vi "LabVIEW_MQTT_Toolkit_V2.vi"() -> ()   [LabVIEW 2021] (continued)
                w5573 = T14 2 items=["User Home"=0, "User Desktop"=1, "User Documents"=2, "User Application Data"=3, "User Preferences"=4, "User Temporary"=5, "Public Documents"=6, "Public Application Data"=7, "Public Preferences"=8, "Public Cache"=13, "System Core Libraries"=9, "System Installed Libraries"=10, "Application Files"=11, "Boot Volume Root"=12] ("system directory type")
                n2249 = Search and Replace String(replace all?=TRUE ("replace all? (F)"), input string=w5568, search string="/") -> (result string=w5589:string)  [unwired: 5 in, 3 out]
                n2250 = Concatenate Strings(w5566, "TimeStamp;Measure Ch_X(g);Ch_Y(g);INC_X(Deg);INC_Y(Deg)", "\n") -> (w5582:string)
                n2251 = Concatenate Strings(w5589, "_" ("string"), "S_E_T.csv") -> (w5590:string)
                n2252 = call <vilib>:"Get System Directory.vi"("system directory type"=w5573) -> ("system directory"=w5583:path)  [unwired: 10 in]
                n2253 = Decimate 1D Array(w5606) -> (w5605:dbl[], w5603:dbl[], w5601:dbl[], w5602:dbl[])
                n2254 = for {
                  tunnel: [w5637] -> w5600 mode=indexing
                  tunnel: w5604 -> [w5631] mode=indexing
                  tunnel: w5605 -> [w5628] mode=indexing
                  tunnel: w5603 -> [w5627] mode=indexing
                  tunnel: w5601 -> [w5626] mode=indexing
                  tunnel: w5602 -> [w5625] mode=indexing
                  tunnel: [w5628] -> w5599 mode=indexing
                  tunnel: [w5627] -> w5598 mode=indexing
                  tunnel: [w5626] -> w5597 mode=indexing
                  tunnel: [w5625] -> w5596 mode=indexing
                  tunnel: w5595 -> [w5620]
                  tunnel: w5594 -> [w5619]
                  tunnel: w5593 -> [w5618] mode=indexing
                  tunnel: w5592 -> [w5617]
                  tunnel: [w5612] -> w5591
                  n2255 = Join Numbers(hi=w5620, lo=w5619) -> ((hi.lo)=w5622:u32)
                  n2256 = To Double Precision Float(number=w5618) -> (double precision float=w5623:dbl)
                  n2257 = Number To Decimal String(number=w5631) -> (decimal integer string=w5636:string)  [unwired: 1 in]
                  n2258 = Number To Fractional String(number=w5628, precision (6)=i16 3 ("width (-)")) -> (F-format string=w5638:string)  [unwired: 2 in]
                  n2259 = Number To Fractional String(number=w5627, precision (6)=i16 3 ("width (-)")) -> (F-format string=w5634:string)  [unwired: 2 in]
                  n2260 = Number To Fractional String(number=w5626, precision (6)=i16 3 ("width (-)")) -> (F-format string=w5632:string)  [unwired: 2 in]
                  n2261 = Number To Fractional String(number=w5625, precision (6)=i16 3 ("width (-)")) -> (F-format string=w5629:string)  [unwired: 2 in]
                  n2262 = Build Array(w5636, w5638, w5634, w5632, w5629) -> (w5637:string[])
                  n2263 = Divide(x=w5623, y=w5617) -> (x/y=w5624:dbl)
                  n2264 = To Unsigned Quad Integer(1:w5622) -> (0:w5621:u64)
                  n2265 = call "Unix Time to Timestamp.vi"("Fractional Second"=w5624, "Unix Time (s)"=w5621) -> ("Timestamp"=w5611:timestamp)  [unwired: 8 in, 1 out]
                  n2266 = Format Date/Time String(seconds (now)=w5611, UTC format=TRUE) -> (date/time string=w5613:string)  [unwired: 1 in]
                  n2267 = Scan From String(format string="%<%x %H:%M:%S%3u>T", input string=w5613) -> (output 1=w5614:timestamp)  [unwired: 3 in, 3 out]
                  n2268 = To Double Precision Float(number=w5614) -> (double precision float=w5612:dbl)
                }
                n2269 = Build Path(base path=w5583, name or relative path="Logfile") -> (appended path=w5584:path)
                n2270 = call <vilib>:"Check if File or Folder Exists.vi"("path"=w5584) -> ("file or folder exists?"=w5585:bool, "dup path"=w5586:path)  [unwired: 8 in, 1 out]
                n2271 = case shown="False" w5585 {
                  tunnel: w5586 -> [w5609 w5610]
                  tunnel: [w5608 w5610] -> w5587
                  frame False {
                    n2272 = Create Folder(path (use dialog)=w5609) -> (created path=w5608:path)  [unwired: 2 in, 2 out]
                  }
                  frame True {
                  }
                }
                n2273 = Build Path(base path=w5587, name or relative path=w5590) -> (appended path=w5588:path)
                n2274 = Open/Create/Replace File(file path (use dialog)=w5588, operation (0:open)=T11."open or create") -> (refnum out=w5581:refnum<file>, error out=w5579:errorcluster)  [unwired: 4 in, 1 out]
                n2275 = Write to Text File(file (use dialog)=w5581, text=w5582, error in=w5579) -> (refnum out=w5580:refnum<file>, error out=w5578:errorcluster)  [unwired: 1 in, 1 out]
                n2276 = Close File(refnum=w5580, error in=w5578) -> (path=w5567:path)  [unwired: 1 out]
              }
              frame 31 {
                w5647 = T14 2 items=["User Home"=0, "User Desktop"=1, "User Documents"=2, "User Application Data"=3, "User Preferences"=4, "User Temporary"=5, "Public Documents"=6, "Public Application Data"=7, "Public Preferences"=8, "Public Cache"=13, "System Core Libraries"=9, "System Installed Libraries"=10, "Application Files"=11, "Boot Volume Root"=12] ("system directory type")
                n2277 = Search and Replace String(replace all?=TRUE ("replace all? (F)"), input string=w5642, search string="/") -> (result string=w5663:string)  [unwired: 5 in, 3 out]
                n2278 = Concatenate Strings(w5640, "TimeStamp;Measure Ch_Z(g);Ch_X(g);Ch_Y(g);INC_X(Deg);INC_Y(Deg)", "\n") -> (w5656:string)
                n2279 = Concatenate Strings(w5663, "_" ("string"), "S_E_T.csv") -> (w5664:string)
                n2280 = call <vilib>:"Get System Directory.vi"("system directory type"=w5647) -> ("system directory"=w5657:path)  [unwired: 10 in]
                n2281 = Decimate 1D Array(w5682) -> (w5681:dbl[], w5680:dbl[], w5679:dbl[], w5678:dbl[], w5676:dbl[])
                n2282 = for {
                  tunnel: [w5716] -> w5675 mode=indexing
                  tunnel: w5677 -> [w5710] mode=indexing
                  tunnel: w5681 -> [w5705] mode=indexing
                  tunnel: w5680 -> [w5704] mode=indexing
                  tunnel: w5679 -> [w5703] mode=indexing
                  tunnel: w5678 -> [w5702] mode=indexing
                  tunnel: w5676 -> [w5701] mode=indexing
                  tunnel: [w5705] -> w5674 mode=indexing
                  tunnel: [w5704] -> w5673 mode=indexing
                  tunnel: [w5703] -> w5672 mode=indexing
                  tunnel: [w5702] -> w5671 mode=indexing
                  tunnel: [w5701] -> w5670 mode=indexing
                  tunnel: w5669 -> [w5696]
                  tunnel: w5668 -> [w5695]
                  tunnel: w5667 -> [w5694] mode=indexing
                  tunnel: w5666 -> [w5693]
                  tunnel: [w5687] -> w5665
                  n2283 = Join Numbers(hi=w5696, lo=w5695) -> ((hi.lo)=w5698:u32)
                  n2284 = To Double Precision Float(number=w5694) -> (double precision float=w5699:dbl)
                  n2285 = Number To Decimal String(number=w5710) -> (decimal integer string=w5715:string)  [unwired: 1 in]
                  n2286 = Number To Fractional String(number=w5705, precision (6)=i16 3 ("width (-)")) -> (F-format string=w5717:string)  [unwired: 2 in]
                  n2287 = Number To Fractional String(number=w5704, precision (6)=i16 3 ("width (-)")) -> (F-format string=w5713:string)  [unwired: 2 in]
                  n2288 = Number To Fractional String(number=w5703, precision (6)=i16 3 ("width (-)")) -> (F-format string=w5711:string)  [unwired: 2 in]
                  n2289 = Number To Fractional String(number=w5702, precision (6)=i16 3 ("width (-)")) -> (F-format string=w5708:string)  [unwired: 2 in]
                  n2290 = Number To Fractional String(number=w5701, precision (6)=i16 3 ("width (-)")) -> (F-format string=w5706:string)  [unwired: 2 in]
                  n2291 = Build Array(w5715, w5717, w5713, w5711, w5708, w5706) -> (w5716:string[])
                  n2292 = Divide(x=w5699, y=w5693) -> (x/y=w5700:dbl)
                  n2293 = To Unsigned Quad Integer(1:w5698) -> (0:w5697:u64)
                  n2294 = call "Unix Time to Timestamp.vi"("Fractional Second"=w5700, "Unix Time (s)"=w5697) -> ("Timestamp"=w5688:timestamp)  [unwired: 8 in, 1 out]
                  n2295 = Format Date/Time String(seconds (now)=w5688, UTC format=TRUE) -> (date/time string=w5689:string)  [unwired: 1 in]
                  n2296 = Scan From String(format string="%<%x %H:%M:%S%3u>T", input string=w5689) -> (output 1=w5690:timestamp)  [unwired: 3 in, 3 out]
                  n2297 = To Double Precision Float(number=w5690) -> (double precision float=w5687:dbl)
                }
                n2298 = Build Path(base path=w5657, name or relative path="Logfile") -> (appended path=w5658:path)
                n2299 = call <vilib>:"Check if File or Folder Exists.vi"("path"=w5658) -> ("file or folder exists?"=w5659:bool, "dup path"=w5660:path)  [unwired: 8 in, 1 out]
                n2300 = case shown="False" w5659 {
                  tunnel: w5660 -> [w5685 w5686]
                  tunnel: [w5684 w5686] -> w5661
                  frame False {
                    n2301 = Create Folder(path (use dialog)=w5685) -> (created path=w5684:path)  [unwired: 2 in, 2 out]
                  }
                  frame True {
                  }
                }
                n2302 = Build Path(base path=w5661, name or relative path=w5664) -> (appended path=w5662:path)
                n2303 = Open/Create/Replace File(file path (use dialog)=w5662, operation (0:open)=T11."open or create") -> (refnum out=w5655:refnum<file>, error out=w5653:errorcluster)  [unwired: 4 in, 1 out]
                n2304 = Write to Text File(file (use dialog)=w5655, text=w5656, error in=w5653) -> (refnum out=w5654:refnum<file>, error out=w5652:errorcluster)  [unwired: 1 in, 1 out]
                n2305 = Close File(refnum=w5654, error in=w5652) -> (path=w5641:path)  [unwired: 1 out]
              }
            }
            "Enabled channels" <- w3579
            "CH_Z Graph" <- w3501
            "CH_X Graph" <- w3499
            "CH_Y Graph" <- w3498
            "INC_X Graph" <- w3497
            "INC_Y Graph" <- w3496
            "File path" <- w3488
            n2306 = property on="CH_Z Graph" class="WFChart (strict)"("XScale.Offset"=w3491) -> ()  [unwired: 2 in, 2 out]
            n2307 = property on="INC_Y Graph" class="WFChart (strict)"("XScale.Offset"=w3487) -> ()  [unwired: 2 in, 2 out]
            n2308 = property on="CH_Y Graph" class="WFChart (strict)"("XScale.Offset"=w3490) -> ()  [unwired: 2 in, 2 out]
            n2309 = property on="CH_X Graph" class="WFChart (strict)"("XScale.Offset"=w3441) -> ()  [unwired: 2 in, 2 out]
            n2310 = property on="INC_X Graph" class="WFChart (strict)"("XScale.Offset"=w3489) -> ()  [unwired: 2 in, 2 out]
            n2311 = call-poly <vilib>:"Write Delimited Spreadsheet.vi"("file path (dialog if empty)"=w3488, "format (%s)"="%s", "2D data"=w3503, "append to file? (new file:F)"=TRUE, "transpose? (no:F)"=FALSE, "delimiter (\\t)"=";" ("delimiter (\\t)")) -> ()  [unwired: 8 in, 2 out]
          }
          frame 7 {
            w5764 = "NA"
            w5800 = T14 2 items=["User Home"=0, "User Desktop"=1, "User Documents"=2, "User Application Data"=3, "User Preferences"=4, "User Temporary"=5, "Public Documents"=6, "Public Application Data"=7, "Public Preferences"=8, "Public Cache"=13, "System Core Libraries"=9, "System Installed Libraries"=10, "Application Files"=11, "Boot Volume Root"=12] ("system directory type")
            # "function to write data in log file"
            # "this block conttain measures + dates of different  sensor channels"
            # "logfile path"
            # "logfile headers"
            # "this block contain Channels bitmap"
            n2312 = String To Byte Array(string=w5907) -> (unsigned byte array=w5841:u8[])
            n2313 = property on="Measure mode" class="Str"() -> ("Value"=w5730:string)  [unwired: 2 in, 2 out]
            n2314 = Array Size(array=w5841) -> (size(s)=w5843:i32)
            n2315 = Array To Cluster(array=w5841) -> (cluster=w5906:T18)
            n2316 = Subtract(x=w5843, y=35) -> (x-y=w5842:i32)
            n2317 = call <vilib>:"Get System Directory.vi"("system directory type"=w5800) -> ("system directory"=w5807:path)  [unwired: 10 in]
            n2318 = String Subset(string=w5755, offset (0)=0, length (rest)=16 ("length (rest)")) -> (substring=w5754:string)
            n2319 = Equal?(x=w5730, y="S_E_T") -> (x = y?=w5732:bool)
            n2320 = Array Subset(array=w5841, index=36, length=w5842) -> (w5743:u8[])
            n2321 = property on="concatenated string" class="Str"() -> ("Value"=w5729:string)  [unwired: 2 in, 2 out]
            n2322 = property on="Measure mode" class="Str"() -> ("Value"=w5726:string)  [unwired: 2 in, 2 out]
            n2323 = Unbundle(w5906) -> ("unsigned byte array[2]"=w5749:u8, "unsigned byte array[3]"=w5905:u8, "unsigned byte array[4]"=w5904:u8, "unsigned byte array[5]"=w5898:u8, "unsigned byte array[6]"=w5897:u8, "unsigned byte array[7]"=w5896:u8, "unsigned byte array[8]"=w5895:u8, "unsigned byte array[9]"=w5894:u8, "unsigned byte array[10]"=w5893:u8, "unsigned byte array[12]"=w5892:u8, "unsigned byte array[16]"=w5889:u8, "unsigned byte array[17]"=w5886:u8, "unsigned byte array[18]"=w5885:u8, "unsigned byte array[19]"=w5873:u8, "unsigned byte array[20]"=w5884:u8, "unsigned byte array[21]"=w5883:u8, "unsigned byte array[22]"=w5882:u8, "unsigned byte array[23]"=w5881:u8, "unsigned byte array[24]"=w5880:u8, "unsigned byte array[25]"=w5890:u8, "unsigned byte array[26]"=w5879:u8, "unsigned byte array[27]"=w5878:u8, "unsigned byte array[28]"=w5871:u8, "unsigned byte array[29]"=w5877:u8, "unsigned byte array[30]"=w5876:u8, "unsigned byte array[31]"=w5875:u8, "unsigned byte array[32]"=w5891:u8, "unsigned byte array[33]"=w5874:u8, "unsigned byte array[34]"=w5887:u8, "unsigned byte array[35]"=w5888:u8)  [unwired: 6 out]
            n2324 = Join Numbers(hi=w5904, lo=w5905) -> ((hi.lo)=w5903:u16)
            n2325 = Join Numbers(hi=w5897, lo=w5898) -> ((hi.lo)=w5902:u16)
            n2326 = Join Numbers(hi=w5894, lo=w5895) -> ((hi.lo)=w5900:u16)
            n2327 = Join Numbers(hi=w5886, lo=w5889) -> ((hi.lo)=w5872:u16)
            n2328 = Join Numbers(hi=w5880, lo=w5881) -> ((hi.lo)=w5866:u16)
            n2329 = Join Numbers(hi=w5879, lo=w5890) -> ((hi.lo)=w5870:u16)
            n2330 = Join Numbers(hi=w5874, lo=w5891) -> ((hi.lo)=w5867:u16)
            n2331 = Join Numbers(hi=w5888, lo=w5887) -> ((hi.lo)=w5741:u16)
            "Number of data per channel" <- w5741
            n2332 = To Unsigned Byte Integer(number=w5892) -> (unsigned 8bit integer=w5753:u8)
            n2333 = case shown="1001" w5753 {
              tunnel: ["" "no active channel" "chZ " "chX " "chZ & chX " "chY " "chZ & chY  " "chX & chY " "chZ& chX& chY " "INC_X " "chZ & INC_X " "chX & INC_X " "chZ& chX & INC_X " "chY & INC_X " "chZ  & chY & INC_X " "chX  & chY & INC_X " "chZ& chX  & chY & INC_X " "INC_Y  " " chZ & INC_Y " " chX & INC_Y  " "chZ & chX & INC_Y " " chY & INC_Y " "chZ & chY & INC_Y" "chX & chY & INC_Y" " chZ &chX & chY & INC_Y  " " INC_X & INC_Y " "chZ &   INC_X & INC_Y" "chX & INC_X & INC_Y" " chZ & chX &  INC_X & INC_Y  " " chY &  INC_X & INC_Y  " "chZ & chY &  INC_X & INC_Y " "chX & chY &  INC_X & INC_Y" "chZ & chX & chY &  INC_X & INC_Y"] -> w5752
              frame Default {
              }
              frame 0 {
              }
              frame 1 {
              }
              frame 2 {
              }
              frame 3 {
              }
              frame 4 {
              }
              frame 5 {
              }
              frame 6 {
              }
              frame 7 {
              }
              frame 8 {
              }
              frame 9 {
              }
              frame 10 {
              }
              frame 11 {
              }
              frame 12 {
              }
              frame 13 {
              }
              frame 14 {
              }
              frame 15 {
              }
              frame 16 {
              }
              frame 17 {
              }
              frame 18 {
              }
              frame 19 {
              }
              frame 20 {
              }
              frame 21 {
              }
              frame 22 {
              }
              frame 23 {
              }
              frame 24 {
              }
              frame 25 {
              }
              frame 26 {
              }
              frame 27 {
              }
              frame 28 {
              }
              frame 29 {
              }
              frame 30 {
              }
              frame 31 {
              }
            }
            "Enabled channels" <- w5752
            n2334 = Join Numbers(hi=w5893, lo=w5900) -> ((hi.lo)=w5899:u32)
            n2335 = Join Numbers(hi=w5896, lo=w5902) -> ((hi.lo)=w5901:u32)
            n2336 = To Word Integer(number=w5903) -> (16bit integer=w5742:i16)
            "Acquisition frequency" <- w5742
            n2337 = To Long Integer(number=w5901) -> (32bit integer=→"Acquisition cycle":i32)
            n2338 = Format Into String(format string="%02d/%02d/%d %02d:%02d:%02d,%d", w5873, w5885, w5872, w5884, w5883, w5882, w5866) -> (resulting string=w5722:string)  [unwired: 2 in, 1 out]
            "Start date" <- w5722
            n2339 = Format Into String(format string="%02d/%02d/%d %02d:%02d:%02d,%d", w5871, w5878, w5870, w5877, w5876, w5875, w5867) -> (resulting string=w5719:string)  [unwired: 2 in, 1 out]
            "End date" <- w5719
            n2340 = Equal?(x=w5726, y="Shock Detection ") -> (x = y?=w5727:bool)
            n2341 = Select(t=w5730, s=w5732, f=w5729) -> (s? t:f=w5725:string)
            n2342 = To Long Integer(number=w5899) -> (32bit integer=→"Acquisition duration":i32)
            n2343 = Build Path(base path=w5807, name or relative path="Logfile") -> (appended path=w5808:path)
            n2344 = call <vilib>:"Check if File or Folder Exists.vi"("path"=w5808) -> ("file or folder exists?"=w5809:bool, "dup path"=w5810:path)  [unwired: 8 in, 1 out]
            n2345 = case shown="False" w5809 {
              tunnel: w5810 -> [w5952 w5953]
              tunnel: [w5951 w5953] -> w5811
              frame False {
                n2346 = Create Folder(path (use dialog)=w5952) -> (created path=w5951:path)  [unwired: 2 in, 2 out]
              }
              frame True {
              }
            }
            n2347 = case shown="7" w5749 {
              tunnel: ["" "LDCDA mode" "Alarm mode" "Streaming mode" "S.E.T mode " "Dynamic mode"] -> w5748
              frame Default {
              }
              frame 1 {
              }
              frame 2 {
              }
              frame 3 {
              }
              frame 6 {
              }
              frame 7 {
              }
            }
            "Acquisition Mode" <- w5748
            n2348 = Select(t=w5726, s=w5727, f=w5725) -> (s? t:f=w5724:string)
            n2349 = Concatenate Strings("Start Date;End Date;Ch_Z_Min value date;Ch_Z_Min value;Ch_Z_Max value date;Ch_Z_Max value;Ch_Z_Average value;Ch_X_Min value date;Ch_X_Min value;Ch_X_Max value date;Ch_X_Max value;Ch_X_Average value;Ch_Y_Min value date;Ch_Y_Min value;Ch_Y_Max value date;Ch_Y_Max value;Ch_Y_Average value;INC_X_Min value date;INC_X_Min value_Deg;INC_X_Max value date;INC_X_Max value_Deg;INC_X_Average value_Deg;INC_Y_Min value date\t;INC_Y_Min value_Deg;INC_Y_Max value date;INC_Y_Max value_Deg;INC_Y_Average value\t", "\n") -> (w5806:string)
            n2350 = Concatenate Strings(w5754, "_" ("string"), w5724, "_" ("string"), "Transmit_Math_Mode.txt") -> (w5813:string)
            n2351 = Build Path(base path=w5811, name or relative path=w5813) -> (appended path=w5812:path)
            n2352 = Open/Create/Replace File(file path (use dialog)=w5812, operation (0:open)=T11."open or create") -> (refnum out=w5805:refnum<file>, error out=w5803:errorcluster)  [unwired: 4 in, 1 out]
            n2353 = Write to Text File(file (use dialog)=w5805, text=w5806, error in=w5803) -> (refnum out=w5804:refnum<file>, error out=w5802:errorcluster)  [unwired: 1 in, 1 out]
            n2354 = Close File(refnum=w5804, error in=w5802) -> (path=w5796:path)  [unwired: 1 out]
            "File path" <- w5796
            n2355 = Decimate 1D Array(w5743) -> (w5865:u8[], w5864:u8[], w5863:u8[], w5862:u8[], w5861:u8[], w5860:u8[], w5859:u8[], w5858:u8[], w5857:u8[], w5856:u8[], w5855:u8[], w5854:u8[], w5853:u8[], w5852:u8[], w5851:u8[], w5850:u8[], w5849:u8[], w5848:u8[], w5847:u8[], w5846:u8[], w5845:u8[])
            n2356 = for {
              tunnel: w5741 -> [w5988]
              tunnel: w5865 -> [w6021] mode=indexing
              tunnel: w5864 -> [w6020] mode=indexing
              tunnel: w5863 -> [w6019] mode=indexing
              tunnel: w5862 -> [w6018] mode=indexing
              tunnel: w5861 -> [w6017] mode=indexing
              tunnel: w5860 -> [w6016] mode=indexing
              tunnel: w5859 -> [w6015] mode=indexing
              tunnel: w5858 -> [w6014] mode=indexing
              tunnel: w5857 -> [w5978] mode=indexing
              tunnel: w5856 -> [w6013] mode=indexing
              tunnel: w5855 -> [w6012] mode=indexing
              tunnel: w5854 -> [w6011] mode=indexing
              tunnel: w5853 -> [w6010] mode=indexing
              tunnel: w5852 -> [w6009] mode=indexing
              tunnel: w5851 -> [w6008] mode=indexing
              tunnel: w5850 -> [w6007] mode=indexing
              tunnel: w5849 -> [w6006] mode=indexing
              tunnel: w5848 -> [w5976] mode=indexing
              tunnel: w5847 -> [w6005] mode=indexing
              tunnel: w5846 -> [w6004] mode=indexing
              tunnel: w5845 -> [w5977] mode=indexing
              tunnel: [w5964] -> w5829 mode=indexing
              tunnel: [w6003] -> w5830 mode=indexing
              tunnel: [w5965] -> w5838 mode=indexing
              tunnel: w5722 -> [w5960]
              tunnel: w5742 -> [w5990]
              tunnel: [w5966] -> w5836 mode=indexing
              tunnel: [w5970] -> w5833 mode=indexing
              tunnel: w5722 -> [w5957]
              tunnel: w5719 -> [w5956]
              tunnel: [w5955] -> w5721
              n2357 = Join Numbers(hi=w6018, lo=w6019) -> ((hi.lo)=w6033:u16)
              n2358 = Join Numbers(hi=w6020, lo=w6021) -> ((hi.lo)=w6034:u16)
              n2359 = Join Numbers(hi=w6010, lo=w6011) -> ((hi.lo)=w6030:u16)
              n2360 = Join Numbers(hi=w6012, lo=w6013) -> ((hi.lo)=w6031:u16)
              n2361 = Join Numbers(hi=w6006, lo=w6007) -> ((hi.lo)=w5982:u16)
              n2362 = Join Numbers(hi=w6004, lo=w6005) -> ((hi.lo)=w6029:u16)
              n2363 = Sign(1:w5978) -> (0:w6032:u8)
              n2364 = To Byte Integer(number=w6014) -> (8bit integer=w5974:i8)
              n2365 = To Byte Integer(number=w6015) -> (8bit integer=w5975:i8)
              n2366 = Sign(1:w5976) -> (0:w5981:u8)
              n2367 = Sign(1:w5977) -> (0:w6028:u8)
              n2368 = Join Numbers(hi=w6016, lo=w6017) -> ((hi.lo)=w6026:u16)
              "index minval" <- w6026
              n2369 = Join Numbers(hi=w6008, lo=w6009) -> ((hi.lo)=w6022:u16)
              "index maxval" <- w6022
              n2370 = Concatenate Strings(w5957, ";", w5956) -> (w5955:string)
              n2371 = Join Numbers(hi=w5974, lo=w5975) -> ((hi.lo)=w5987:u16)
              n2372 = Join Numbers(hi=w6033, lo=w6034) -> ((hi.lo)=w6027:u32)
              "fid min ch1" <- w6027
              n2373 = Join Numbers(hi=w6030, lo=w6031) -> ((hi.lo)=w6023:u32)
              "fid max ch1" <- w6023
              n2374 = To Byte Integer(number=w5981) -> (8bit integer=w5979:i8)
              n2375 = To Word Integer(number=w5982) -> (16bit integer=w5983:i16)
              n2376 = To Byte Integer(number=w6028) -> (8bit integer=w5985:i8)
              n2377 = To Word Integer(number=w6029) -> (16bit integer=w5984:i16)
              n2378 = Scan From String(format string="%<%x %H:%M:%S%3u>T", input string=w5960) -> (output 1=w5995:timestamp)  [unwired: 3 in, 3 out]
              n2379 = Multiply(x=w5988, y=w6027) -> (x*y=w6025:u32)
              n2380 = Multiply(x=w5988, y=w6023) -> (x*y=w6024:u32)
              n2381 = case shown="1" w5979 {
                tunnel: w5983 -> [_ w6043 w6049]
                tunnel: [_ w6041 w6048] -> w5964
                frame Default {
                }
                frame 1 {
                  n2382 = Equal?(x=w6043, y=i16 0) -> (x = y?=w6045:bool)
                  n2383 = Divide(x=w6043, y=-1000.0) -> (x/y=w6042:dbl)
                  n2384 = Select(t=0.0 ("f"), s=w6045, f=w6042) -> (s? t:f=w6041:dbl)
                }
                frame 0 {
                  n2385 = Equal?(x=w6049, y=i16 -1) -> (x = y?=w6052:bool)
                  n2386 = Divide(x=w6049, y=1000.0) -> (x/y=w6050:dbl)
                  n2387 = Select(t=0.0 ("f"), s=w6052, f=w6050) -> (s? t:f=w6048:dbl)
                }
              }
              n2388 = case shown="0" w5985 {
                tunnel: [_ w6036 w6039] -> w6003
                tunnel: w5984 -> [_ w6035 w6038]
                frame Default {
                }
                frame 1 {
                  n2389 = Divide(x=w6035, y=-1000.0) -> (x/y=w6036:dbl)
                }
                frame 0 {
                  n2390 = Divide(x=w6038, y=1000.0) -> (x/y=w6039:dbl)
                }
              }
              n2391 = To Byte Integer(number=w6032) -> (8bit integer=w5980:i8)
              n2392 = To Word Integer(number=w5987) -> (16bit integer=w5986:i16)
              n2393 = case shown="0" w5980 {
                tunnel: w5986 -> [_ w6060 w6065]
                tunnel: [_ w6057 w6064] -> w5965
                frame Default {
                }
                frame 1 {
                  n2394 = Equal?(x=w6060, y=i16 -1) -> (x = y?=w6058:bool)
                  n2395 = Divide(x=w6060, y=-1000.0) -> (x/y=w6055:dbl)
                  n2396 = Select(t=0.0 ("f"), s=w6058, f=w6055) -> (s? t:f=w6057:dbl)
                }
                frame 0 {
                  n2397 = Equal?(x=w6065, y=i16 -1) -> (x = y?=w6066:bool)
                  n2398 = Divide(x=w6065, y=1000.0) -> (x/y=w6062:dbl)
                  n2399 = Select(t=0.0 ("f"), s=w6066, f=w6062) -> (s? t:f=w6064:dbl)
                }
              }
              n2400 = Add(x=w6026, y=w6025) -> (x+y=w5992:u32)
              n2401 = Add(x=w6022, y=w6024) -> (x+y=w5994:u32)
              n2402 = Divide(x=1, y=w5990) -> (x/y=w5997:dbl)
              n2403 = Divide(x=1, y=w5990) -> (x/y=w6000:dbl)
              n2404 = Multiply(x=w5997, y=w5992) -> (x*y=w5998:dbl)
              n2405 = Multiply(x=w6000, y=w5994) -> (x*y=w6001:dbl)
              n2406 = call "Timestamp to Unix Time.vi"("Timestamp (now)"=w5995) -> ("Unix Time (s)"=w6002:i64)  [unwired: 9 in, 1 out]
              n2407 = Add(x=w6002, y=w5998) -> (x+y=w5996:dbl)
              n2408 = Add(x=w6002, y=w6001) -> (x+y=w5999:dbl)
              n2409 = call "Unix Time to Timestamp.vi"("Unix Time (s)"=w5996) -> ("Timestamp"=w5973:timestamp)  [unwired: 9 in, 1 out]
              n2410 = call "Unix Time to Timestamp.vi"("Unix Time (s)"=w5999) -> ("Timestamp"=w5967:timestamp)  [unwired: 9 in, 1 out]
              n2411 = Format Date/Time String(seconds (now)=w5973, UTC format=TRUE) -> (date/time string=w5971:string)  [unwired: 1 in]
              n2412 = Format Date/Time String(seconds (now)=w5967, UTC format=TRUE) -> (date/time string=w5968:string)  [unwired: 1 in]
              n2413 = Equal To 0?(x=w5964) -> (x = 0?=w5962:bool)
              n2414 = Equal To 0?(x=w5965) -> (x = 0?=w5963:bool)
              n2415 = And(x=w5963, y=w5962) -> (x .and. y?=w5961:bool)
              n2416 = Select(t="NA", s=w5961, f=w5971) -> (s? t:f=w5970:string)
              n2417 = Select(t="NA", s=w5961, f=w5968) -> (s? t:f=w5966:string)
            }
            "Max value" <- w5829
            "Average value" <- w5830
            "Min value" <- w5838
            "Min date" <- w5833
            "Max date" <- w5836
            n2418 = Equal?(x=w5793, y=u8 1) -> (x = y?=w5744:bool)
            n2419 = Array To Cluster(array=w5833) -> (cluster=w5834:T19)
            n2420 = Array To Cluster(array=w5838) -> (cluster=w5837:T20)
            n2421 = Array To Cluster(array=w5836) -> (cluster=w5835:T19)
            n2422 = Array To Cluster(array=w5829) -> (cluster=w5832:T20)
            n2423 = Array To Cluster(array=w5830) -> (cluster=w5831:T20)
            n2424 = Equal?(x=w5793, y=u8 6) -> (x = y?=w5720:bool)
            n2425 = Unbundle(w5834) -> ("[0]"=w5740:string, "[1]"=w5825:string, "[2]"=w5822:string, "[3]"=w5738:string, "[4]"=w5737:string)
            n2426 = Unbundle(w5837) -> ("[0]"=w5739:dbl, "[1]"=w5747:dbl, "[2]"=w5821:dbl, "[3]"=w5783:dbl, "[4]"=w5782:dbl)
            n2427 = Unbundle(w5835) -> ("[0]"=w5828:string, "[1]"=w5824:string, "[2]"=w5787:string, "[3]"=w5736:string, "[4]"=w5735:string)
            n2428 = Unbundle(w5832) -> ("[0]"=w5827:dbl, "[1]"=w5820:dbl, "[2]"=w5819:dbl, "[3]"=w5781:dbl, "[4]"=w5780:dbl)
            n2429 = Unbundle(w5831) -> ("[0]"=w5826:dbl, "[1]"=w5823:dbl, "[2]"=w5818:dbl, "[3]"=w5779:dbl, "[4]"=w5778:dbl)
            n2430 = Not Or(1:w5720, 2:w5744) -> (0:w5777:bool)
            n2431 = Number To Fractional String(number=w5783, precision (6)=i16 3 ("width (-)")) -> (F-format string=w5776:string)  [unwired: 2 in]
            n2432 = Number To Fractional String(number=w5781, precision (6)=i16 3 ("width (-)")) -> (F-format string=w5774:string)  [unwired: 2 in]
            n2433 = Number To Fractional String(number=w5779, precision (6)=i16 3 ("width (-)")) -> (F-format string=w5772:string)  [unwired: 2 in]
            n2434 = Number To Fractional String(number=w5782, precision (6)=i16 3 ("width (-)")) -> (F-format string=w5775:string)  [unwired: 2 in]
            n2435 = Number To Fractional String(number=w5780, precision (6)=i16 3 ("width (-)")) -> (F-format string=w5773:string)  [unwired: 2 in]
            n2436 = Number To Fractional String(number=w5778, precision (6)=i16 3 ("width (-)")) -> (F-format string=w5771:string)  [unwired: 2 in]
            n2437 = Select(t=w5737, s=w5777, f="") -> (s? t:f=w5786:string)
            n2438 = Select(t=w5735, s=w5777, f="") -> (s? t:f=w5790:string)
            n2439 = Select(t=w5738, s=w5777, f="NA") -> (s? t:f=w5789:string)
            n2440 = Select(t=w5736, s=w5777, f="NA") -> (s? t:f=w5788:string)
            n2441 = Select(t=w5776, s=w5777, f=w5764) -> (s? t:f=w5770:string)
            n2442 = Select(t=w5774, s=w5777, f=w5764) -> (s? t:f=w5768:string)
            n2443 = Select(t=w5772, s=w5777, f=w5764) -> (s? t:f=w5765:string)
            n2444 = Select(t=w5775, s=w5777, f=w5764) -> (s? t:f=w5769:string)
            n2445 = Select(t=w5773, s=w5777, f=w5764) -> (s? t:f=w5767:string)
            n2446 = Select(t=w5771, s=w5777, f=w5764) -> (s? t:f=w5766:string)
            n2447 = Format Into String(format string=";%S ;%.3f;%s;%.3f;%.3f;%S;%.3f;%s;%.3f;%.3f;%S ;%.3f ;%s;%.3f; %.3f ;%s ;%s; %s ;%s ;%s; %s ;%s ;%s ;%s ;%s\\n", initial string=w5721, w5740, w5739, w5828, w5827, w5826, w5825, w5747, w5824, w5820, w5823, w5822, w5821, w5787, w5819, w5818, w5789, w5770, w5788, w5768, w5765, w5786, w5769, w5790, w5767, w5766) -> (resulting string=w5816:string)  [unwired: 1 in, 1 out]
            n2448 = Build Array(w5816) -> (w5815:string[])
            n2449 = call-poly <vilib>:"Write Delimited Spreadsheet.vi"("file path (dialog if empty)"=w5796, "1D data"=w5815, "append to file? (new file:F)"=TRUE, "transpose? (no:F)"=TRUE, "delimiter (\\t)"=";" ("delimiter (\\t)")) -> ()  [unwired: 9 in, 2 out]
            "Device type" <- w5908
            "String" <- "Ch_Z                    Ch_X                     Ch_Y                     INC_X                     INC_Y" ("String")
          }
        }
        "Measure mode" <- w195
        "Date & time" <- w190
        "Sensor Label" <- w193
        "Device type" <- w194
        "Date & time" <- w190
        "Sensor label" <- w193
        "Measure mode" <- w195
        "Measure" <- w180
        "Measure" <- w180
        "Numeric" <- w175
      }
      event "Data acq .mode": Value Change {
        # "this block is used to disable and enable sampling rate according to the mode of acquisition"
        n2450 = event-data() -> ()  [unwired: 1 in, 1 out]
        n2451 = property on="Data acq .mode" class="Ring (strict)"() -> ("Value"=w6077:u8)  [unwired: 2 in, 2 out]
        n2452 = case shown="3" w6077 {
          tunnel: "Device type" -> [_ w6084 _ w6095 _ _ _]
          frame 2 {
            (unwired) i32[] [1, 2, 3, 4, 5, 6, 7, 8, 9, 10, 11, 12, 13, 14, 15, 16, 17, 18, 19, 20, 21] ("Disabled Items []")
            w6080 = T10."Enabled" ("Disabled")
            w6079 = T10."Disabled and Grayed Out" ("Disabled")
            n2453 = property on="Streaming options" class="RadioBtnsControl (strict)"("DisabledEnum"=w6079) -> ()  [unwired: 2 in, 2 out]
            n2454 = property on="Data Acq duration" class="Clust (strict)"("DisabledEnum"=w6079) -> ()  [unwired: 2 in, 2 out]
            n2455 = property on="Math notif ratio" class="DigNum (strict)"("DisabledEnum"=w6080) -> ()  [unwired: 2 in, 2 out]
            n2456 = property on="Tx ratio" class="DigNum (strict)"("DisabledEnum"=w6080) -> ()  [unwired: 2 in, 2 out]
            n2457 = property on="Data acq cycle/Notif cycle" class="Clust (strict)"("DisabledEnum"=w6080) -> ()  [unwired: 2 in, 2 out]
            n2458 = property on="Sampling rate" class="Ring (strict)"("DisabledEnum"=w6079) -> ()  [unwired: 2 in, 2 out]
          }
          frame 3 {
            w6082 = T10."Enabled" ("Disabled")
            w6083 = T10."Disabled and Grayed Out" ("Disabled")
            n2459 = property on="Tx ratio" class="DigNum (strict)"("DisabledEnum"=w6083) -> ()  [unwired: 2 in, 2 out]
            n2460 = property on="Data Acq duration" class="Clust (strict)"("DisabledEnum"=w6083) -> ()  [unwired: 2 in, 2 out]
            n2461 = property on="Math notif ratio" class="DigNum (strict)"("DisabledEnum"=w6083) -> ()  [unwired: 2 in, 2 out]
            n2462 = property on="Data acq cycle/Notif cycle" class="Clust (strict)"("DisabledEnum"=w6083) -> ()  [unwired: 2 in, 2 out]
            n2463 = case shown="1" w6084 {
              frame Default {
              }
              frame 1 {
                n2464 = property on="Sampling rate" class="Ring (strict)"("Disabled Items []"=i32[] [1, 2, 3, 5, 6, 8, 9, 11, 12, 13, 14, 15, 17, 19, 21]) -> ()  [unwired: 2 in, 2 out]
              }
              frame 2 {
                n2465 = property on="Sampling rate" class="Ring (strict)"("Disabled Items []"=i32[] []) -> ()  [unwired: 2 in, 2 out]
              }
              frame 3 {
                n2466 = property on="Sampling rate" class="Ring (strict)"("Disabled Items []"=i32[] []) -> ()  [unwired: 2 in, 2 out]
              }
              frame 4 {
                n2467 = property on="Sampling rate" class="Ring (strict)"("Disabled Items []"=i32[] []) -> ()  [unwired: 2 in, 2 out]
              }
              frame 5 {
                n2468 = property on="Sampling rate" class="Ring (strict)"("Disabled Items []"=i32[] []) -> ()  [unwired: 2 in, 2 out]
              }
              frame 0 {
                n2469 = property on="Sampling rate" class="Ring (strict)"("Disabled Items []"=i32[] []) -> ()  [unwired: 2 in, 2 out]
              }
            }
            n2470 = property on="Sampling rate" class="Ring (strict)"("DisabledEnum"=w6082) -> ()  [unwired: 2 in, 2 out]
            n2471 = property on="Streaming options" class="RadioBtnsControl (strict)"("DisabledEnum"=w6082) -> ()  [unwired: 2 in, 2 out]
            n2472 = property on="Sampling rate" class="Ring (strict)"("Disabled Items []"=i32[] []) -> ()  [unwired: 2 in, 2 out]
          }
          frame 4 {
            w6092 = T10."Enabled" ("Disabled")
            w6091 = T10."Disabled and Grayed Out" ("Disabled")
            n2473 = property on="Data Acq duration" class="Clust (strict)"("DisabledEnum"=w6091) -> ()  [unwired: 2 in, 2 out]
            n2474 = property on="Streaming options" class="RadioBtnsControl (strict)"("DisabledEnum"=w6091) -> ()  [unwired: 2 in, 2 out]
            n2475 = property on="Sampling rate" class="Ring (strict)"("DisabledEnum"=w6091) -> ()  [unwired: 2 in, 2 out]
            n2476 = property on="Math notif ratio" class="DigNum (strict)"("DisabledEnum"=w6091) -> ()  [unwired: 2 in, 2 out]
            n2477 = property on="Tx ratio" class="DigNum (strict)"("DisabledEnum"=w6092) -> ()  [unwired: 2 in, 2 out]
            n2478 = property on="Data acq cycle/Notif cycle" class="Clust (strict)"("DisabledEnum"=w6092) -> ()  [unwired: 2 in, 2 out]
            n2479 = property on="Sampling rate" class="Ring (strict)"("DisabledEnum"=w6091) -> ()  [unwired: 2 in, 2 out]
          }
          frame 5 {
            w6093 = T10."Enabled" ("Disabled")
            w6094 = T10."Disabled and Grayed Out" ("Disabled")
            n2480 = property on="Tx ratio" class="DigNum (strict)"("DisabledEnum"=w6094) -> ()  [unwired: 2 in, 2 out]
            n2481 = property on="Streaming options" class="RadioBtnsControl (strict)"("DisabledEnum"=w6094) -> ()  [unwired: 2 in, 2 out]
            n2482 = property on="Data acq cycle/Notif cycle" class="Clust (strict)"("DisabledEnum"=w6093) -> ()  [unwired: 2 in, 2 out]
            n2483 = property on="Math notif ratio" class="DigNum (strict)"("DisabledEnum"=w6094) -> ()  [unwired: 2 in, 2 out]
            n2484 = property on="Sampling rate" class="Ring (strict)"("Disabled Items []"=i32[] [14, 15, 16, 17, 18, 19, 20, 21]) -> ()  [unwired: 2 in, 2 out]
            n2485 = property on="Sampling rate" class="Ring (strict)"("DisabledEnum"=w6093) -> ()  [unwired: 2 in, 2 out]
            n2486 = property on="Data Acq duration" class="Clust (strict)"("DisabledEnum"=w6093) -> ()  [unwired: 2 in, 2 out]
            n2487 = case shown="Default" w6095 {
              frame Default {
              }
              frame 1 {
                n2488 = property on="Sampling rate" class="Ring (strict)"("Disabled Items []"=i32[] [1, 2, 3, 5, 6, 8, 9, 11, 12, 13, 14, 15, 16, 17, 18, 19, 20, 21]) -> ()  [unwired: 2 in, 2 out]
              }
              frame 2 {
                n2489 = property on="Sampling rate" class="Ring (strict)"("Disabled Items []"=i32[] [14, 15, 16, 17, 18, 19, 20, 21]) -> ()  [unwired: 2 in, 2 out]
              }
              frame 3 {
                n2490 = property on="Sampling rate" class="Ring (strict)"("Disabled Items []"=i32[] [14, 15, 16, 17, 18, 19, 20, 21]) -> ()  [unwired: 2 in, 2 out]
              }
              frame 4 {
                n2491 = property on="Sampling rate" class="Ring (strict)"("Disabled Items []"=i32[] [14, 15, 16, 17, 18, 19, 20, 21]) -> ()  [unwired: 2 in, 2 out]
              }
              frame 5 {
                n2492 = property on="Sampling rate" class="Ring (strict)"("Disabled Items []"=i32[] [14, 15, 16, 17, 18, 19, 20, 21]) -> ()  [unwired: 2 in, 2 out]
              }
              frame 0 {
                n2493 = property on="Sampling rate" class="Ring (strict)"("Disabled Items []"=i32[] [14, 15, 16, 17, 18, 19, 20, 21]) -> ()  [unwired: 2 in, 2 out]
              }
            }
          }
          frame 6 {
            w6104 = T10."Enabled" ("Disabled")
            w6105 = T10."Disabled and Grayed Out" ("Disabled")
            n2494 = property on="Sampling rate" class="Ring (strict)"("DisabledEnum"=w6104) -> ()  [unwired: 2 in, 2 out]
            n2495 = property on="Math notif ratio" class="DigNum (strict)"("DisabledEnum"=w6105) -> ()  [unwired: 2 in, 2 out]
            n2496 = property on="Data Acq duration" class="Clust (strict)"("DisabledEnum"=w6104) -> ()  [unwired: 2 in, 2 out]
            n2497 = property on="Data acq cycle/Notif cycle" class="Clust (strict)"("DisabledEnum"=w6104) -> ()  [unwired: 2 in, 2 out]
            n2498 = property on="Tx ratio" class="DigNum (strict)"("DisabledEnum"=w6105) -> ()  [unwired: 2 in, 2 out]
            n2499 = property on="Streaming options" class="RadioBtnsControl (strict)"("DisabledEnum"=w6105) -> ()  [unwired: 2 in, 2 out]
            n2500 = property on="Sampling rate" class="Ring (strict)"("Disabled Items []"=i32[] [1, 2, 3, 5, 6, 8, 9, 11, 12, 13, 14, 15, 17, 19, 21]) -> ()  [unwired: 2 in, 2 out]
          }
          frame Default {
          }
          frame 1 {
            w6106 = T10."Enabled" ("Disabled")
            n2501 = property on="Streaming options" class="RadioBtnsControl (strict)"("DisabledEnum"=w6106) -> ()  [unwired: 2 in, 2 out]
            n2502 = property on="Tx ratio" class="DigNum (strict)"("DisabledEnum"=w6106) -> ()  [unwired: 2 in, 2 out]
            n2503 = property on="Data acq cycle/Notif cycle" class="Clust (strict)"("DisabledEnum"=w6106) -> ()  [unwired: 2 in, 2 out]
            n2504 = property on="Data Acq duration" class="Clust (strict)"("DisabledEnum"=w6106) -> ()  [unwired: 2 in, 2 out]
            n2505 = property on="Math notif ratio" class="DigNum (strict)"("DisabledEnum"=w6106) -> ()  [unwired: 2 in, 2 out]
            n2506 = property on="Sampling rate" class="Ring (strict)"("DisabledEnum"=w6106) -> ()  [unwired: 2 in, 2 out]
          }
        }
      }
      event "Streaming options": Value Change {
        # "used to enable and disable Data acq duration and data acq cycle according to the selected mode"
        n2507 = event-data() -> ()  [unwired: 1 in, 1 out]
        n2508 = case shown="\"One Shot\"" "Streaming options" {
          frame "No Selection", Default {
          }
          frame "Continuous Monitoring" {
            w6109 = T10."Disabled and Grayed Out" ("Disabled")
            n2509 = property on="Data Acq duration" class="Clust (strict)"("DisabledEnum"=w6109) -> ()  [unwired: 2 in, 2 out]
            n2510 = property on="Data acq cycle/Notif cycle" class="Clust (strict)"("DisabledEnum"=w6109) -> ()  [unwired: 2 in, 2 out]
          }
          frame "Burst" {
            w6110 = T10."Enabled" ("Disabled")
            n2511 = property on="Data acq cycle/Notif cycle" class="Clust (strict)"("DisabledEnum"=w6110) -> ()  [unwired: 2 in, 2 out]
            n2512 = property on="Data Acq duration" class="Clust (strict)"("DisabledEnum"=w6110) -> ()  [unwired: 2 in, 2 out]
          }
          frame "One Shot" {
            n2513 = property on="Data acq cycle/Notif cycle" class="Clust (strict)"("DisabledEnum"=T10."Disabled and Grayed Out" ("Disabled")) -> ()  [unwired: 2 in, 2 out]
            n2514 = property on="Data Acq duration" class="Clust (strict)"("DisabledEnum"=T10."Enabled" ("Disabled")) -> ()  [unwired: 2 in, 2 out]
          }
        }
      }
      event "Math notif ratio": Value Change {
        n2515 = event-data() -> ()  [unwired: 1 in, 6 out]
        n2516 = property on="Math notif ratio" class="DigNum (strict)"() -> ("Value"=w6113:u16)  [unwired: 2 in, 2 out]
        n2517 = Greater?(x=w6113, y=u16 2427) -> (0:w6117:bool)
        n2518 = Less?(x=w6113, y=u16 2) -> (x < y?=w6118:bool)
        n2519 = Or(x=w6117, y=w6118) -> (x .or. y?=w6116:bool)
        n2520 = case shown="False" w6116 {
          frame False {
          }
          frame True {
            n2521 = One Button Dialog(message="Math Notif.ratio should be between 2 and 2427", button name ("OK")="OK") -> ()  [unwired: 1 out]
          }
        }
      }
      event "Tx ratio": Value Change {
        n2522 = event-data() -> ()  [unwired: 1 in, 1 out]
        n2523 = property on="Tx ratio" class="DigNum (strict)"() -> ("Value"=w6122:u8)  [unwired: 2 in, 2 out]
        n2524 = Greater?(x=w6122, y=u8 9) -> (0:w6127:bool)
        n2525 = Less?(x=w6122, y=u8 1) -> (x < y?=w6126:bool)
        n2526 = Or(x=w6127, y=w6126) -> (x .or. y?=w6125:bool)
        n2527 = case shown="False" w6125 {
          frame False {
          }
          frame True {
            n2528 = One Button Dialog(message="TX_RATIO  must be within following range[1,9].", button name ("OK")="OK") -> ()  [unwired: 1 out]
          }
        }
      }
    }
  }
  n2529 = Unregister For Events(event registration refnum=w3, error in=w5) -> (error out=w4:errorcluster)
  n2530 = call "api_mqttDisconnect.vi"("error in (no error)"=w4) -> ("error out"=w10:errorcluster)  [unwired: 13 in, 1 out]
  n2531 = call "mqttTXdataQueue.vi"("function"=mqttTXdataQueueFunction."deinit", "error in (no error)"=w10) -> ("error out"=w6:errorcluster)  [unwired: 12 in, 1 out]
  n2532 = call "mqttRXsubscriptionEvent.vi"("function"=mqttRXsubscriptionEventFunction."deinit", "error in (no error)"=w6) -> ()  [unwired: 12 in, 2 out]
